vi "BL_GetErrorMsg.vi"(8 "error in (no error)":errorcluster, 10 "Error Code":i32, 11 "Potentiostat Galvanostat in":refnum<class "Potentiostat Galvanostat.lvclass">) -> (0 "error out":errorcluster, 1 "Error Message":string, 2 "Error Code":i32, 3 "Potentiostat Galvanostat out":refnum<class "Potentiostat Galvanostat.lvclass">)   [LabVIEW 2018, in "Potentiostat Galvanostat.lvclass"]
doc: "This function tests the communication speed between the library and the selected channel. \nNOTE: This function is for advanced user only."
uses:
  Potentiostat Galvanostat.lvclass
  Potentiostat Galvanostat.lvclass/Potentiostat Galvanostat.ctl
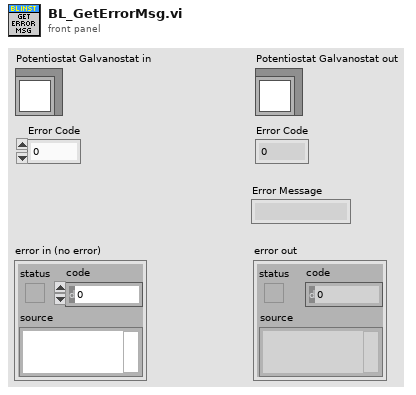
[diagram p1: front panel]
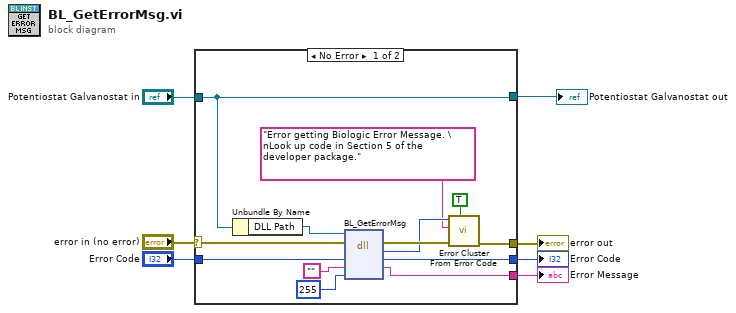
[diagram p0: block diagram]
diagram:
  n1 = case shown="No Error" "error in (no error)" {
    selector: "error in (no error)" -> [w11 w21]
    tunnel: [w17 w21] -> w7
    tunnel: [w16 _] -> w6
    tunnel: [w8 _] -> w5
    tunnel: "Error Code" -> [w14 _]
    tunnel: "Potentiostat Galvanostat in" -> [w10 w22]
    tunnel: [w10 w22] -> w1
    frame No Error {
      n2 = Unbundle By Name(w10) -> ("DLL Path"=w12:path)
      n3 = dll-call lib="C:/Projects/LabVIEW/BioLogic Instrument Driver/libs/EC-Lab Development Package/EClib.*" fn="BL_GetErrorMsg"(path in=w12, error in=w11, "Error Code"=w14, "Error Message"="", "Size"=u32 255) -> (error out=w20:errorcluster, "Error Message Error Code"=w19:i32, "Error Code"=w16:i32, "Error Message"=w8:string)  [unwired: 2 in, 1 out]
      n4 = call <vilib>:"Error Cluster From Error Code.vi"("show call chain? (False)"=TRUE, "error in (no error)"=w20, "error message (\"\")"="Error getting Biologic Error Message. \nLook up code in Section 5 of the developer package." ("t"), "error code (0)"=w19) -> ("error out"=w17:errorcluster)  [unwired: 5 in]
    }
    frame Error {
    }
  }
  "error out" <- w7
  "Potentiostat Galvanostat out" <- w1
  "Error Code" <- w6
  "Error Message" <- w5
